vi "CAN_F2C_Logger.vi"() -> ()   [LabVIEW 2015]
uses:
  Type Def Controls/CAN Message & Channels.ctl
  Type Def Controls/CAN Channel.ctl
  <vilib>/FPGAPlugInAG/cRIO-9114/niLvFpga_Open_cRIO-9114.vi
  <vilib>/rvi/interface/common/dynamic/niFpgaDynamicAddResources.vi
  <vilib>/Utility/error.llb/Error Cluster From Error Code.vi
  <vilib>/rvi/errors/niLvFpgaAdjustHostInterfaceError.vi
  <vilib>/FPGAPlugInAG/Dynamic/niLvFpga_Close_Dynamic.vi
  <vilib>/rvi/interface/nirviOpenFPGA/nirviOpenFPGA.xnode
  FPGA Bitfiles/Canlogger3CHConv_FPGATarget_CANFrameFeedwith_OKF8Z1gjNso.lvbitx
  FPGA/CAN Frame Feed with Overflow Control (FPGA).vi
  <vilib>/rvi/interface/nirviReadWriteControl/nirviReadWriteControl.xnode
  <vilib>/rvi/interface/nirviMethod/nirviMethod.xnode
  <vilib>/rvi/interface/nirviCloseFPGA/nirviCloseFPGA.xnode
  <vilib>/rvi/errors/niLvFpgaMergeErrorWithErrorCode.vi
  NiFpgaLv.dll
  <vilib>/rvi/interface/Simulation/niFpgaSimulationCallBeginRW.vi
  <vilib>/FPGAPlugInAG/Dynamic/niLvFpga_ReadFifo_Dynamic.vi
panel:
  in  "TDMS file path":path=path "c:/CAN1.tdms"
  out "Message with Ch's Corresponding to Scaled Data":T1 {"Channels"."Mode Channel Config"."Byte Order" items=["Intel", "Motorola"]; "Number of Bytes" max=8 step=1}
  out "Frames Processed":i32
  out "Messages":T1[](array[typedef]) {"Channels"."Mode Channel Config"."Byte Order" items=["Intel", "Motorola"]; "Number of Bytes" max=8 step=1}
  out "Elements Remaining":i32
  in  "Selected Channels Binary File Path":path=path "c:/selected_can_messages.bin"
  out "Frame Processing\nTime Avg (msec)":dbl
  out "Channel Data Arrary Out":dbl[](array[numeric])
  in  "Stop":bool
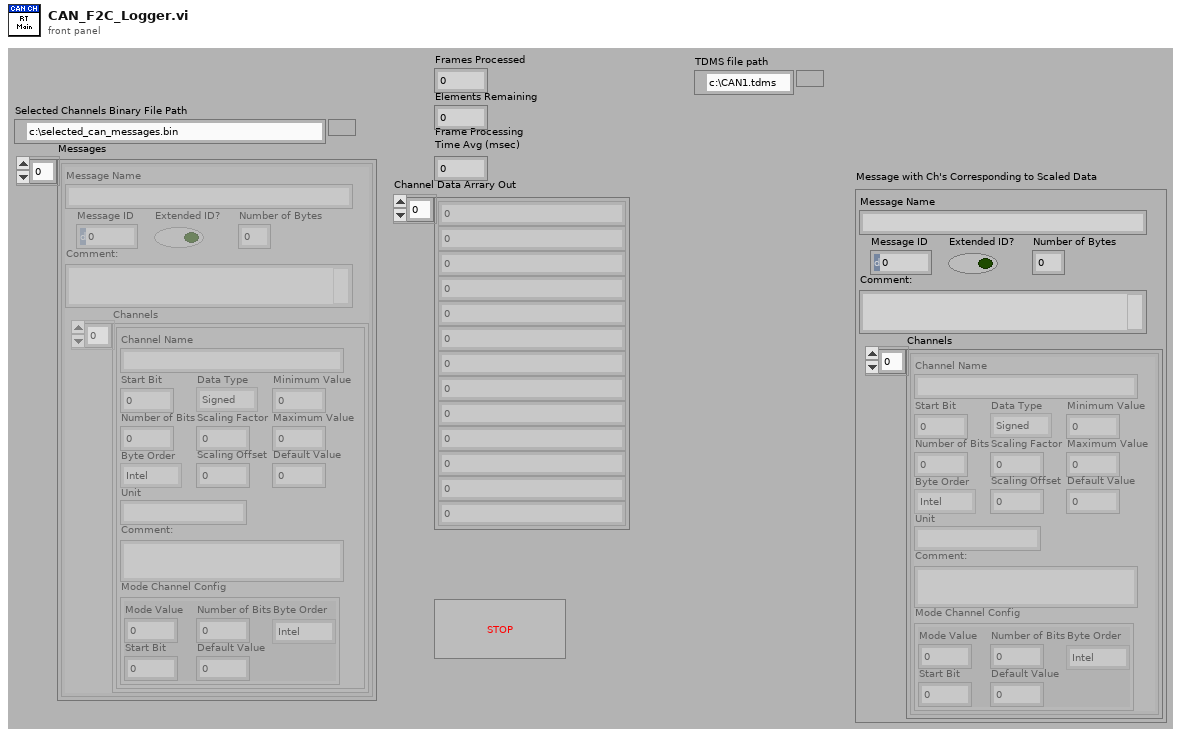
[diagram p1: front panel]
types:
  T1 = typedef "CAN Message & Channels.ctl" = cluster{"Message Name":string, "Message ID":u32, "Extended ID?":bool, "Number of Bytes":u32, "Comment:":string, "Channels":T2[]}
  T2 = typedef "CAN Channel.ctl" = cluster{"Channel Name":string, "Start Bit":u8, "Number of Bits":u8, "Byte Order":enum8{"Intel", "Motorola"}, "Data Type":enum8{"Signed", "Unsigned", "IEEE Float"}, "Scaling Factor":dbl, "Scaling Offset":dbl, "Minimum Value":dbl, "Maximum Value":dbl, "Default Value":dbl, "Unit":string, "Comment:":string, "Mode Channel Config":cluster{"Mode Value":u8, "Start Bit":u8, "Number of Bits":u8, "Default Value":u8, "Byte Order":u8}}
  T3 = enum16{"open", "open or create", "create or replace", "create", "open (read-only)"}
  T4 = typedef "CAN_IO_SJA1000 Acceptance Filter.ctl" = enum8{"Dual", "Single"}
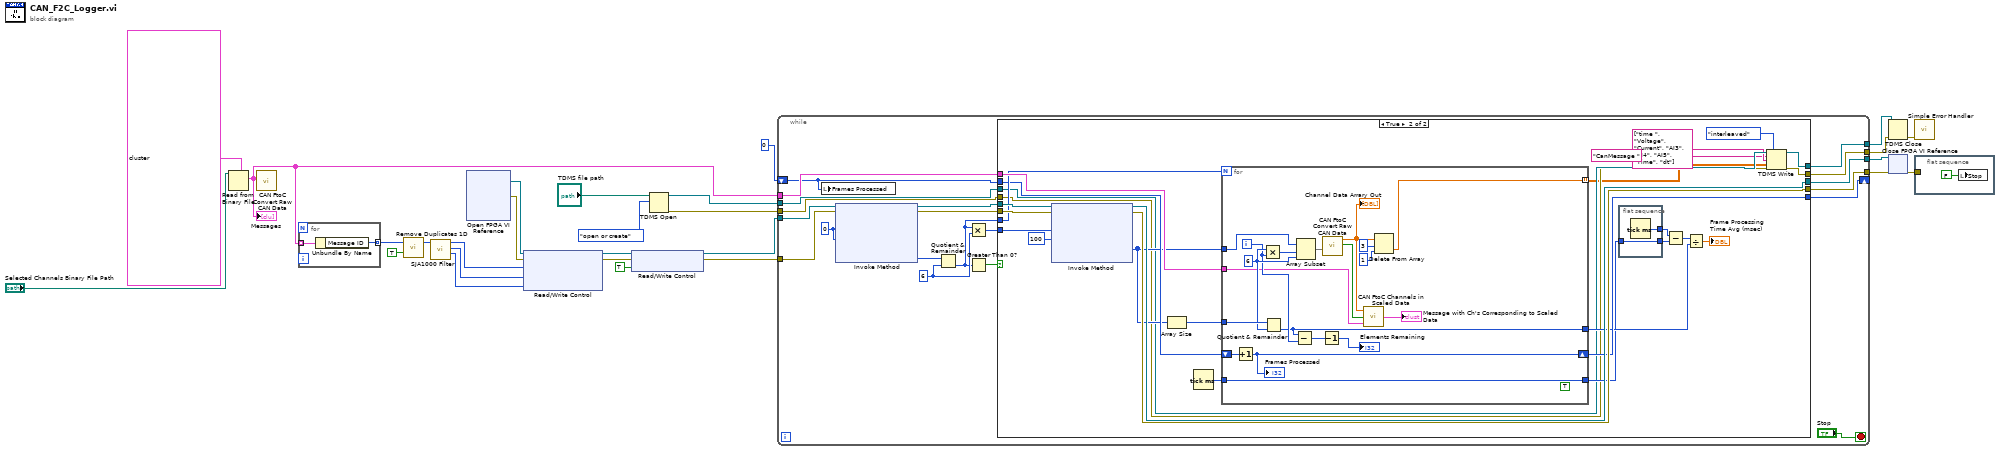
[diagram p0: block diagram]
diagram:
  n1 = Read from Binary File(5:T1[] [{"Message Name"="PATS_Control_Info2006", "Message ID"=65, "Extended ID?"=FALSE, "Number of Bytes"=8, "Comment:"="", "Channels"=[{"Channel Name"="PATS_CONTROL_DATA_VALID", "Start Bit"=12, "Number of Bits"=1, "Byte Order"=enum."Motorola", "Data Type"=enum."Unsigned", "Scaling Factor"=1.0, "Scaling Offset"=0.0, "Minimum Value"=0.0, "Maximum Value"=1.0, "Default Value"=0.0, "Unit"="", "Comment:"="", "Mode Channel Config"={"Mode Value"=0, "Start Bit"=0, "Number of Bits"=0, "Default Value"=0, "Byte Order"=0}}, {"Channel Name"="PATS_CONTROL_SECURITY_TYPE", "Start Bit"=13, "Number of Bits"=1, "Byte Order"=enum."Motorola", "Data Type"=enum."Unsigned", "Scaling Factor"=1.0, "Scaling Offset"=0.0, "Minimum Value"=0.0, "Maximum Value"=1.0, "Default Value"=0.0, "Unit"="", "Comment:"="", "Mode Channel Config"={"Mode Value"=0, "Start Bit"=0, "Number of Bits"=0, "Default Value"=0, "Byte Order"=0}}, {"Channel Name"="PATS_CONTROL_STATUS", "Start Bit"=14, "Number of Bits"=2, "Byte Order"=enum."Motorola", "Data Type"=enum."Unsigned", "Scaling Factor"=1.0, "Scaling Offset"=0.0, "Minimum Value"=0.0, "Maximum Value"=3.0, "Default Value"=0.0, "Unit"="", "Comment:"="", "Mode Channel Config"={"Mode Value"=0, "Start Bit"=0, "Number of Bits"=0, "Default Value"=0, "Byte Order"=0}}]}] ("Messages 2"), 11:"Selected Channels Binary File Path") -> (2:w8:T1[])  [unwired: 4 in, 3 out]
  "Messages" <- w8
  n2 = call "CAN FtoC Convert Raw CAN Data.vi"("Ordered Messages"=w8) -> ()  [unwired: 9 in, 2 out]
  n3 = for {
    tunnel: w8 -> [w28] mode=indexing
    tunnel: [w29] -> w23 mode=indexing
    n4 = Unbundle By Name(w28) -> ("Message ID"=w29:u32)
  }
  n5 = call "Remove Duplicates 1D.vi"("Sort First"=TRUE, "Array IN"=w23) -> ("Array OUT"=w25:u32[])  [unwired: 1 out]
  n6 = call "SJA1000 Filter.vi"("Selected U32 IDs"=w25) -> ("SJA1000 Code"=w13:u32, "SJA1000 Mask"=w14:u32, "SJA1000 Filter Mode"=w15:T4)  [unwired: 7 in, 1 out]
  n7 = xnode "Open FPGA VI Reference"() -> ("FPGA VI Reference Out"=w22:refnum<k20>, "error out"=w16:errorcluster)  [unwired: 2 in]
  n8 = xnode "Read/Write Control"("FPGA VI Reference In"=w22, "error in"=w16, "SJA1000 Filter Mode"=w15, "SJA1000 Filter Mask"=w14, "SJA1000 Filter Code"=w13) -> ("FPGA VI Reference Out"=w21:refnum<k20>, "error out"=w20:errorcluster)
  n9 = xnode "Read/Write Control"("FPGA VI Reference In"=w21, "error in"=w20, "Set Filter and Start"=TRUE) -> ("FPGA VI Reference Out"=w18:refnum<k20>, "error out"=w17:errorcluster)
  n10 = TDMS Open(10:T3."open or create" ("operation (0:open)"), 11:"TDMS file path") -> (0:w5:errorcluster, 3:w6:refnum<k34>)  [unwired: 5 in]
  n11 = while {
    tunnel: w18 -> [w34]
    tunnel: [w48] -> w27
    tunnel: [w47] -> w26
    tunnel: w17 -> [w46]
    tunnel: w8 -> [w37]
    shift-right: [w36] -> _
    shift-left: 0 -> [w35]
    tunnel: w6 -> [w33]
    tunnel: w5 -> [w32]
    tunnel: [w31] -> w4
    tunnel: [w30] -> w3
    stop <- "Stop" stop-if-true
    w41 = u32 6 ("y")
    w43 = u32 0 ("Number of Elements")
    n12 = local write "Frames Processed"(w35) -> ()
    n13 = xnode "Invoke Method"("FPGA VI Reference In"=w34, "error in"=w46, "Number of Elements"=w43, "Timeout (ms)"=w43) -> ("FPGA VI Reference Out"=w45:refnum<k20>, "error out"=w44:errorcluster, "Elements Remaining"=w42:u32)  [unwired: 1 out]
    n14 = Quotient & Remainder(x=w42, y=w41) -> (floor(x/y)=w38:u32)  [unwired: 1 out]
    n15 = Multiply(x=w38, y=w41) -> (x*y=w40:u32)
    n16 = Greater Than 0?(x=w38) -> (x > 0?=w39:bool)
    n17 = case shown="True" w39 {
      tunnel: w37 -> [_ w81]
      tunnel: [w54 w80] -> w48
      tunnel: [w53 w79] -> w47
      tunnel: w45 -> [w54 w78]
      tunnel: w44 -> [w53 w77]
      tunnel: w40 -> [_ w76]
      tunnel: w38 -> [_ w74]
      tunnel: w35 -> [w52 w73]
      tunnel: [w52 w72] -> w36
      tunnel: w33 -> [w50 w60]
      tunnel: w32 -> [w51 w59]
      tunnel: [w50 w63] -> w31
      tunnel: [w51 w62] -> w30
      frame False {
      }
      frame True {
        n18 = xnode "Invoke Method"("FPGA VI Reference In"=w78, "error in"=w77, "Number of Elements"=w76, "Timeout (ms)"=100) -> ("FPGA VI Reference Out"=w80:refnum<k20>, "error out"=w79:errorcluster, "Data"=w61:u32[])  [unwired: 1 out]
        n19 = Array Size(array=w61) -> (size(s)=w71:i32)
        n20 = Tick Count (ms)() -> (millisecond timer value=w68:u32)
        n21 = for {
          N: w74 -> [_]
          tunnel: w81 -> [w90]
          tunnel: w61 -> [w100]
          shift-right: [w98] -> w72
          shift-left: w73 -> [w99]
          tunnel: w71 -> [w97]
          tunnel: [w92] -> w65
          tunnel: w68 -> [w92]
          tunnel: [w91] -> w66
          tunnel: [w84] -> w58 mode=indexing
          i -> [w94]
          (unwired) TRUE ("append to file? (new file:F)")
          w95 = 6 ("x")
          n22 = Increment(x=w99) -> (x+1=w98:i32)
          "Frames Processed" <- w98
          n23 = Multiply(x=w95, y=w94) -> (x*y=w101:i32)
          n24 = Quotient & Remainder(x=w97, y=w95) -> (floor(x/y)=w91:i32)  [unwired: 1 out]
          n25 = Subtract(x=w91, y=w94) -> (x-y=w96:i32)
          n26 = Array Subset(array=w100, index=w101, length=w95) -> (w102:u32[])
          n27 = Decrement(x=w96) -> (x-1=→"Elements Remaining":i32)
          n28 = call "CAN FtoC Convert Raw CAN Data.vi"("Frame Data"=w102) -> ("Ch Array"=w89:bool[], "Channel Data Out"=w85:dbl[])  [unwired: 9 in]
          "Channel Data Arrary Out" <- w85
          n29 = call "CAN FtoC Channels in Scaled Data.vi"("Message Array"=w90, "Ch Array"=w89, "Channel Data Out"=w85) -> ("Message"=→"Message with Ch's Corresponding to Scaled Data":T1)
          n30 = Delete From Array(array=w85, length=3, index=1) -> (deleted portion=w84:dbl[])  [unwired: 1 out]
        }
        n31 = flat-sequence {
          tunnel: [w83] -> w69
          tunnel: w65 -> [w82]
          tunnel: [w82] -> w64
          frame #0 {
            n32 = Tick Count (ms)() -> (millisecond timer value=w83:u32)
          }
        }
        n33 = Subtract(x=w69, y=w64) -> (x-y=w70:u32)
        n34 = Divide(x=w70, y=w66) -> (x/y=→"Frame Processing\nTime Avg (msec)":dbl)
        n35 = TDMS Write(0:w60, 1:enum16{"decimated", "interleaved"}."interleaved" ("data layout (0:decimated)"), 5:"CanMessage " ("group name in (Untitled)"), 7:string[] ["time ", "Voltage", "Current", "AI3", "AI4", "AI5", "Time", "dt"] ("channel name(s) in (Untitled)"), 9:w58, 11:w59) -> (4:w63:refnum<k34>, 15:w62:errorcluster)  [unwired: 2 out]
      }
    }
  }
  n36 = TDMS Close(8:w3, 11:w4) -> (0:w2:errorcluster)  [unwired: 1 out]
  n37 = xnode "Close FPGA VI Reference"("FPGA VI Reference In"=w27, "error in"=w26) -> ("error out"=w11:errorcluster)
  n38 = call <vilib>:"Simple Error Handler.vi"("error in (no error)"=w2) -> ()  [unwired: 4 in, 5 out]
  n39 = flat-sequence {
    tunnel: w11 -> [_]
    frame #0 {
      n40 = local write "Stop"(FALSE ("Stop")) -> ()
    }
  }
